vi "Get MSS.vi"(11 "Series Actor in":refnum<class "Series Actor.lvclass">) -> (2 "Measure and Stimulus Subsystems":refnum<class "MSS.lvclass">, 3 "Series Actor out":refnum<class "Series Actor.lvclass">)   [LabVIEW 2023, in "Series Actor.lvlib" / "Series Actor.lvclass"]
uses:
  Series Actor.lvclass
  HAL/MSS/MSS.lvclass
  Series Actor.lvclass/Series Actor.ctl
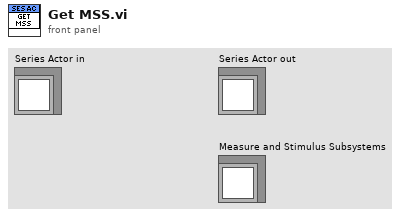
[diagram p1: front panel]
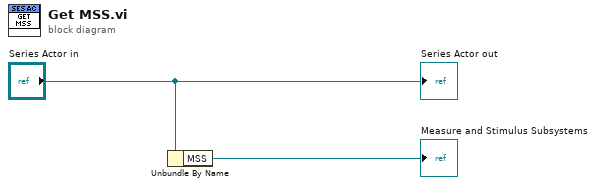
[diagram p0: block diagram]
diagram:
  n1 = Unbundle By Name("Series Actor in") -> ("MSS"=→"Measure and Stimulus Subsystems":refnum<class "MSS.lvclass">)
  "Series Actor out" <- "Series Actor in"
